vi "Read User-Defined States.vi"(8 "error in (no error)":errorcluster, 11 "CSM-Helper in":refnum<class "CSM-Helper.lvclass">) -> (0 "error out":errorcluster, 2 "Array":string[](array[string]), 3 "CSM-Helper out":refnum<class "CSM-Helper.lvclass">)   [LabVIEW 2017, in "CSM-Helper.lvclass"]
doc: "### Read User-Defined States.vi\n\n-- <b>Controls</b> --\n- <b>CSM-Helper in</b>: CSMHelper input\n\n-- <b>Indicators</b> --\n- <b>Array</b>:\n- <b>CSM-Helper out</b>: CSMHelper output"
uses:
  CSM-Helper.lvclass
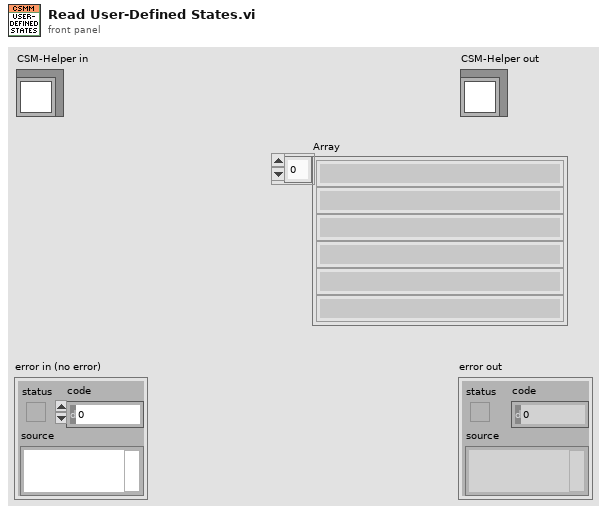
[diagram p1: front panel]
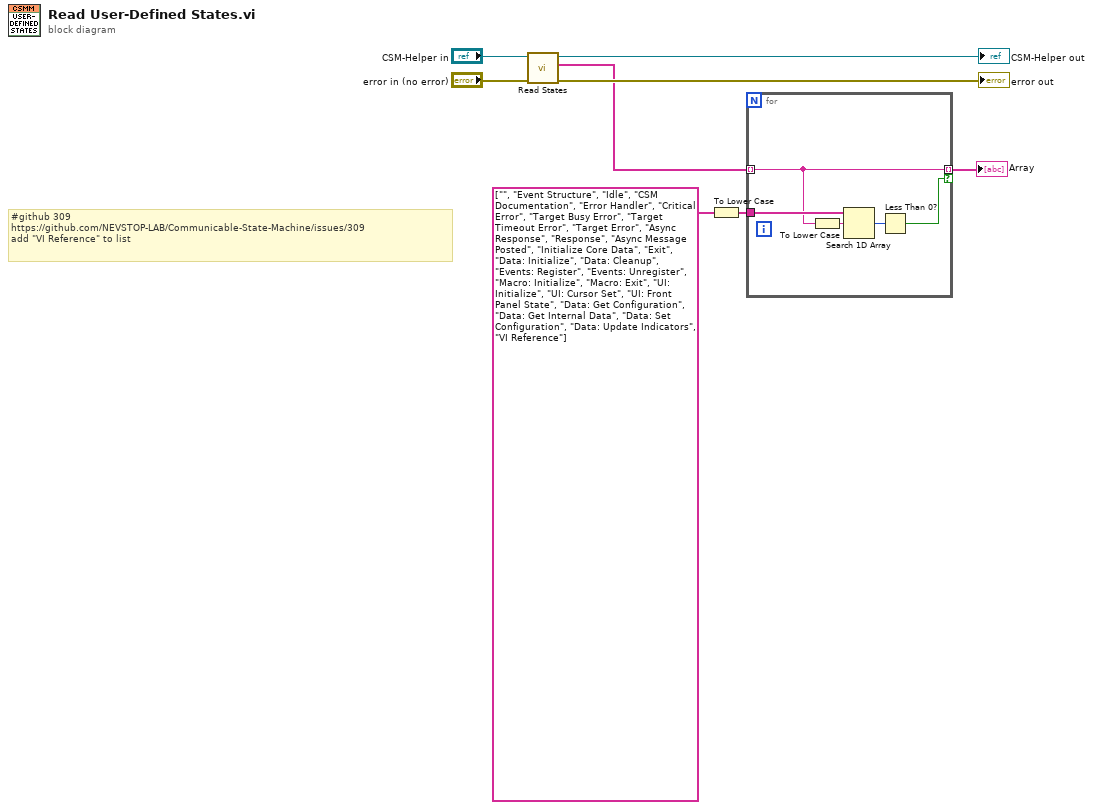
[diagram p0: block diagram]
diagram:
  # "#github 309\nhttps://github.com/NEVSTOP-LAB/Communicable-State-Machine/issues/309\nadd \"VI Reference\" to list"
  n1 = call "Read States.vi"("error in (no error)"="error in (no error)", "CSM-Helper in"="CSM-Helper in") -> ("error out"=→"error out":errorcluster, "Value"=w1:string[], "CSM-Helper out"=→"CSM-Helper out":refnum<class "CSM-Helper.lvclass">)  [unwired: 7 in]
  n2 = To Lower Case(string=string[] ["", "Event Structure", "Idle", "CSM Documentation", "Error Handler", "Critical Error", "Target Busy Error", "Target Timeout Error", "Target Error", "Async Response", "Response", "Async Message Posted", "Initialize Core Data", "Exit", "Data: Initialize", "Data: Cleanup", "Events: Register", "Events: Unregister", "Macro: Initialize", "Macro: Exit", "UI: Initialize", "UI: Cursor Set", "UI: Front Panel State", "Data: Get Configuration", "Data: Get Internal Data", "Data: Set Configuration", "Data: Update Indicators", "VI Reference"] ("items to filter")) -> (all lower case string=w7:string[])
  n3 = for {
    tunnel: w1 -> [w9] mode=indexing
    tunnel: [w9] -> w6 mode=indexing if=w10
    tunnel: w7 -> [w12]
    n4 = To Lower Case(string=w9) -> (all lower case string=w11:string)
    n5 = Search 1D Array(1D array=w12, element=w11) -> (index of element=w13:i32)  [unwired: 1 in]
    n6 = Less Than 0?(x=w13) -> (x < 0?=w10:bool)
  }
  "Array" <- w6
